vi "daq_example_ao_2.vi"() -> ()   [LabVIEW 2015]
uses:
  <vilib>/DAQmx/write.llb/DAQmx Write (Analog 1D DBL 1Chan NSamp).vi
  <vilib>/DAQmx/create/channels.llb/DAQmx Create Channel (AO-Voltage-Basic).vi
  <vilib>/DAQmx/configure/timing.llb/DAQmx Timing (Sample Clock).vi
  <vilib>/DAQmx/miscellaneous.llb/DAQmx Fill In Error Info.vi
  <resource>/objmgr/daqmx.rc
panel:
  in  "Use Sin":bool
  in  "Path":path
  out "number of samples written per channel":u32
  out "Waveform Graph":waveform(dbl)(graph)
  out "error out":errorcluster
  out "SampClk.Rate":dbl
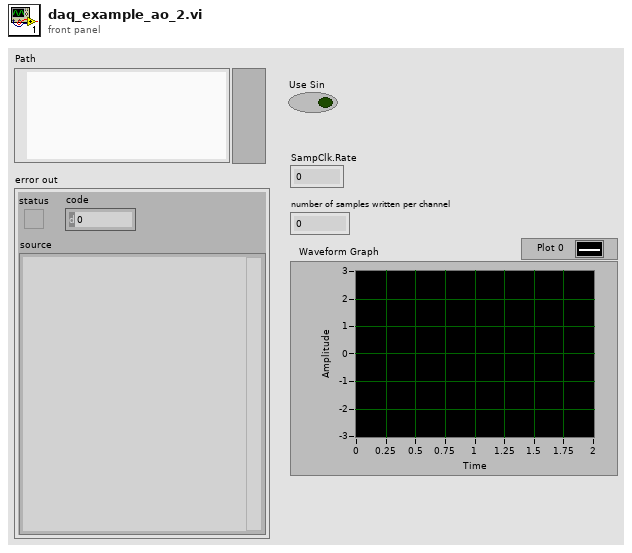
[diagram p1: front panel]
types:
  T1 = cluster{"piezo_command":dbl[], "alignment_command":dbl[]}
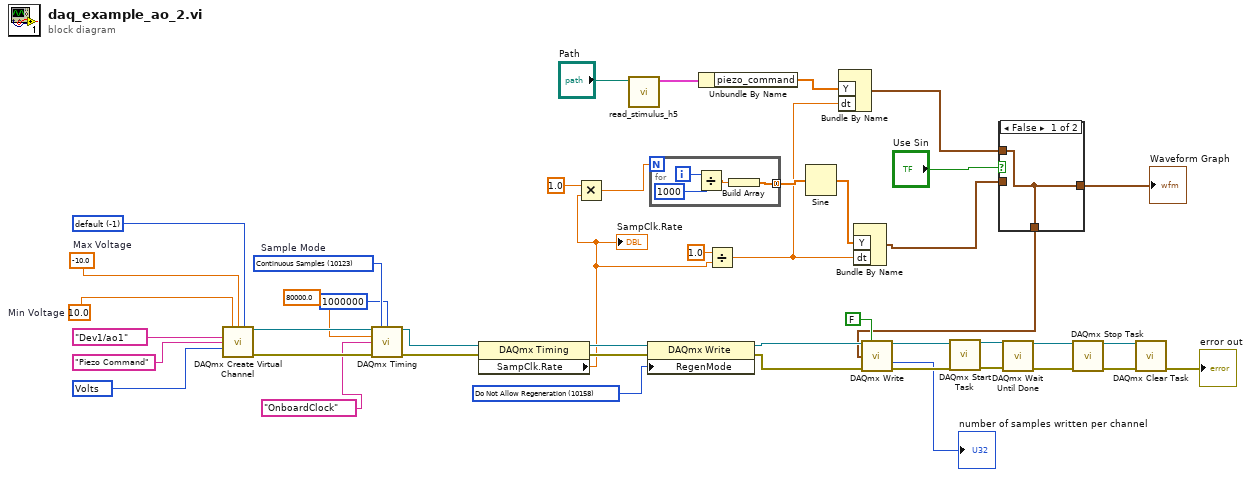
[diagram p0: block diagram]
diagram:
  w45 = 10158 items=["Allow Regeneration"=10097, "Do Not Allow Regeneration"=10158] ("RegenMode")
  w35 = 10123 items=["Finite Samples"=10178, "Continuous Samples"=10123, "Hardware Timed Single Point"=12522]  # Sample Mode
  w42 = -1 items=["default"=-1, "RSE"=10083, "NRSE"=10078, "Differential"=10106, "Pseudodifferential"=12529] ("input terminal configuration")
  w41 = 10348 items=["Volts"=10348, "From Custom Scale"=10065] ("units")
  w38 = 10.0  # Min Voltage
  w39 = -10.0  # Max Voltage
  n1 = call-poly <vilib>:"DAQmx Create Virtual Channel.vi"("maximum value"=w38, "minimum value"=w39, "output terminal configuration"=w42, "physical channels"=tag "Dev1/ao1", "name to assign"="Piezo Command", "units"=w41) -> ("task out"=w36:refnum<k21>, "error out"=w37:errorcluster)  [unwired: 8 in]
  n2 = call-poly <vilib>:"DAQmx Timing.vi"("task/channels in"=w36, "sample mode"=w35, "samples per channel"=1000000, "rate"=80000.0 ("Rate"), "source"=tag "OnboardClock", "error in"=w37) -> ("task out"=w32:refnum<k21>, "error out"=w33:errorcluster)  [unwired: 8 in]
  n3 = property class="DAQmx Timing"(reference=w32, error in=w33) -> (reference out=w43:refnum<k21>, error out=w44:errorcluster, "SampClk.Rate"=w15:dbl)
  "SampClk.Rate" <- w15
  n4 = Multiply(x=1.0, y=w15) -> (x*y=w13:dbl)
  n5 = call "read_stimulus_h5.vi"("Path"="Path") -> ("output cluster"=w10:T1)  [unwired: 7 in, 3 out]
  n6 = property class="DAQmx Write"(reference=w43, error in=w44, "RegenMode"=w45) -> (reference out=w30:refnum<k21>, error out=w29:errorcluster)
  n7 = for {
    N: w13 -> [_]
    tunnel: [w49] -> w18 mode=concatenating
    i -> [w48]
    n8 = Divide(x=w48, y=1000) -> (x/y=w47:dbl)
    n9 = Build Array(w47) -> (w49:dbl[])
  }
  n10 = Unbundle By Name(w10) -> ("piezo_command"=w9:dbl[])
  n11 = Divide(x=1.0, y=w15) -> (x/y=w2:dbl)
  n12 = Sine(x=w18) -> (sin(x)=w17:dbl[])
  n13 = Bundle By Name("Y"=w9, "dt"=w2) -> (w4:waveform(dbl))  [unwired: 1 in]
  n14 = Bundle By Name("Y"=w17, "dt"=w2) -> (w8:waveform(dbl))  [unwired: 1 in]
  n15 = case shown="False" "Use Sin" {
    tunnel: w8 -> [_ w51]
    tunnel: [w50 w51] -> w6
    tunnel: [w50 w51] -> w5
    tunnel: w4 -> [w50 _]
    frame False {
    }
    frame True {
    }
  }
  "Waveform Graph" <- w5
  n16 = call-poly <vilib>:"DAQmx Write.vi"("task/channels in"=w30, "auto start"=FALSE, "data"=w6, "error in"=w29) -> ("task out"=w20:refnum<k21>, "number of samples written per channel"=→"number of samples written per channel":u32, "error out"=w21:errorcluster)  [unwired: 9 in]
  n17 = call <vilib>:"DAQmx Start Task.vi"("task/channels in"=w20, "error in"=w21) -> ("task out"=w23:refnum<k21>, "error out"=w22:errorcluster)  [unwired: 12 in]
  n18 = call <vilib>:"DAQmx Wait Until Done.vi"("task/channels in"=w23, "error in"=w22) -> ("task out"=w28:refnum<k21>, "error out"=w27:errorcluster)  [unwired: 12 in]
  n19 = call <vilib>:"DAQmx Stop Task.vi"("task/channels in"=w28, "error in"=w27) -> ("task out"=w26:refnum<k21>, "error out"=w25:errorcluster)  [unwired: 12 in]
  n20 = call <vilib>:"DAQmx Clear Task.vi"("task in"=w26, "error in"=w25) -> ("error out"=→"error out":errorcluster)  [unwired: 13 in]
